vi "E816_Sample_Application_1.vi"() -> ()   [LabVIEW 2013]
doc: "This VI demonstrates how to initialize an E-816 system, how to move an axis and how to query for the position value of this axis.\n\nIn this example the E-816 is connected through COM port 1 with baudrate 57600. The VI runs E816_Configuration_Setup.vi with these specified settings, moves the first axis relative to its current position, waits for the movement to finish and reads the position of the axis and the error status of the controller. The diagram shows how to combine the driver VIs for these tasks. \n\nFor an example of how to command multiple axes through an USB connection see E816_Sample_ Application_1a.vi\n\nWarning: Before running this VI, modify the interface settings on the block diagram to reflect your configuration. The predefined settings provided with the VI probably do not match your system."
panel:
  in  "stop":bool
  in  "error in":errorcluster
  out "Running":bool caption="Configuration_Setup.vi is running"
  out "error out":errorcluster
  out "Position":dbl[](array[numeric]) format="%.6f"
  out "First conn. axis":string[](array[string])
  out "Identification":string
  # "This VI demonstrates how to initialize an E-816 system, how to move an axis and how to query for the position value of this axis. \nThe VI runs E816_Configuration_Setup.vi with specified settings, moves the first axis relative to its current position and reads the\nposition of this axis. The diagram shows how to combine the driver VIs for these tasks. \n\nWarning: Before running this VI, modify the interface settings on the block diagram to reflect your configuration. The predefined \n                 settings provided with the VI probably do not match your system."
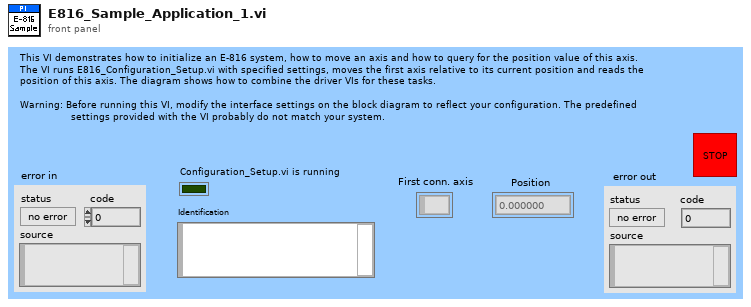
[diagram p1: front panel]
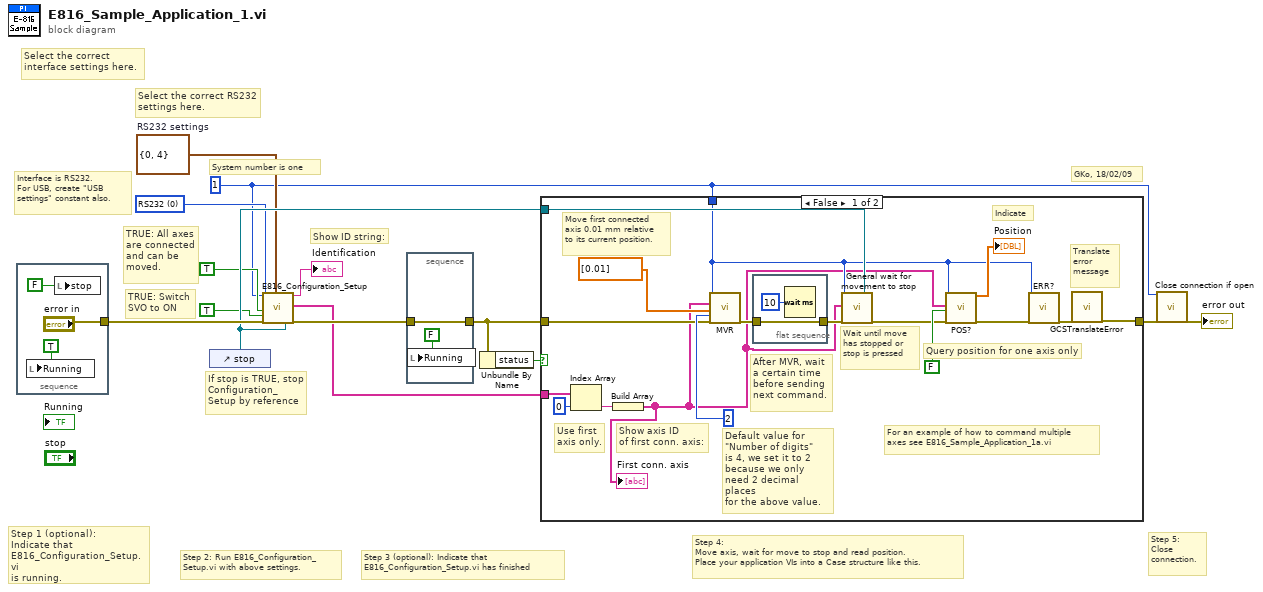
[diagram p0: block diagram]
diagram:
  w4 = u16 0 items=["RS232", "USB"] ("Interface")
  w7 = cluster{"Portnumber":i32, "Baudrate":u16} {"Portnumber"=0, "Baudrate"=4}  # RS232 settings
  w1 = 1 ("System no.")
  # "Select the correct\ninterface settings here."
  # "Step 5: \nClose\nconnection."
  # "Interface is RS232.\nFor USB, create \"USB\nsettings\" constant also."
  # "TRUE: All axes\nare connected\nand can be\nmoved."
  # "TRUE: Switch\nSVO to ON"
  # "If stop is TRUE, stop\nConfiguration_\nSetup by reference"
  # "Step 4: \nMove axis, wait for move to stop and read position.\nPlace your application VIs into a Case structure like this."
  # "Select the correct RS232\nsettings here."
  # "GKo, 18/02/09"
  # "Step 3 (optional): Indicate that \nE816_Configuration_Setup.vi has finished"
  # "Step 2: Run E816_Configuration_\nSetup.vi with above settings."
  # "Step 1 (optional): \nIndicate that \nE816_Configuration_Setup.vi\nis running."
  # "Show ID string:"
  # "System number is one"
  n1 = stacked-sequence {
    tunnel: ["error in"] -> w12
    frame #0 {
      n2 = local write "Running"(TRUE ("Running")) -> ()
      n3 = local write "stop"(FALSE ("stop")) -> ()
    }
  }
  n4 = control-ref of="stop"() -> (w9:refnum<vi>)
  n5 = call "E816_Configuration_Setup.vi"("System no."=w1, "Interface"=w4, "All axes?"=TRUE, "Change servo \nstatus to ON?"=TRUE ("Use dialog to define\nconnected stages?"), "error in"=w12, "RS232 settings"=w7, "Stop refnum"=w9) -> ("Identification"=→"Identification":string, "Conn. Axes"=w8:string[], "error out"=w13:errorcluster)  [unwired: 4 in, 6 out]
  n6 = stacked-sequence {
    tunnel: w13 -> [w19]
    tunnel: [w19] -> w11
    frame #0 {
      n7 = local write "Running"(FALSE ("Running")) -> ()
    }
  }
  n8 = Unbundle By Name(w11) -> ("status"=w10:bool)
  n9 = case shown="False" w10 {
    tunnel: [w31 w39] -> w3
    tunnel: w8 -> [w23 _]
    tunnel: w1 -> [w27 _]
    tunnel: w11 -> [w32 w39]
    tunnel: w9 -> [w30 _]
    frame False {
      # "Show axis ID\nof first conn. axis:"
      # "For an example of how to command multiple\naxes see E816_Sample_Application_1a.vi"
      # "Use first\naxis only."
      # "After MVR, wait\na certain time\nbefore sending\nnext command."
      # "Translate\nerror \nmessage"
      # "Wait until move\nhas stopped or\nstop is pressed"
      # "Indicate"
      # "Default value for\n\"Number of digits\"\nis 4, we set it to 2\nbecause we only\nneed 2 decimal places\nfor the above value."
      # "Move first connected\naxis 0.01 mm relative\nto its current position."
      # "Query position for one axis only"
      n10 = Index Array(array=w23, index=0) -> (element=w21:string)
      n11 = Build Array(w21) -> (w20:string[])
      "First conn. axis" <- w20
      n12 = call "MVR.vi"("System no."=w27, "Axes to move"=w20, "Position values"=dbl[] [0.01], "No.of digits"=i16 2, "error in"=w32) -> ("error out"=w25:errorcluster)  [unwired: 14 out]
      n13 = flat-sequence {
        tunnel: w25 -> [w38]
        tunnel: [w38] -> w24
        frame #0 {
          n14 = Wait (ms)(milliseconds to wait=u32 10) -> ()  [unwired: 1 out]
        }
      }
      n15 = call "General wait for movement to stop.vi"("System no."=w27, "Axes to wait for"=w20, "error in"=w24, "Stop refnum"=w30) -> ("error out"=w26:errorcluster)  [unwired: 4 in, 11 out]
      n16 = call "POS?.vi"("System no."=w27, "Axes to query"=w20, "All axes?"=FALSE, "error in"=w26) -> ("Position"=→"Position":dbl[], "error out"=w29:errorcluster)  [unwired: 1 in, 13 out]
      n17 = call "ERR?.vi"("System no."=w27, "error in"=w29) -> ("error out"=w28:errorcluster)  [unwired: 17 out]
      n18 = call "GCSTranslateError.vi"("error in"=w28) -> ("error out"=w31:errorcluster)  [unwired: 18 out]
    }
    frame True {
      # "Error during initialization"
    }
  }
  n19 = call "Close connection if open.vi"("System no."=w1, "error in"=w3) -> ("error out"=→"error out":errorcluster)  [unwired: 1 in, 16 out]
